vi "Queue - Engine - Main.vi"(6 "timeout in ms (-1)":i32=-1, 7 "Operation":enum16{"Enqueue", "Dequeue", "Flush", "Release"}(ring)=enum."Dequeue", 8 "error in":errorcluster, 10 "Queue Data In":string, 11 "Queue Name In":string) -> (0 "error out":errorcluster, 1 "timed out?":bool, 2 "Data Out":string)   [LabVIEW 2011]
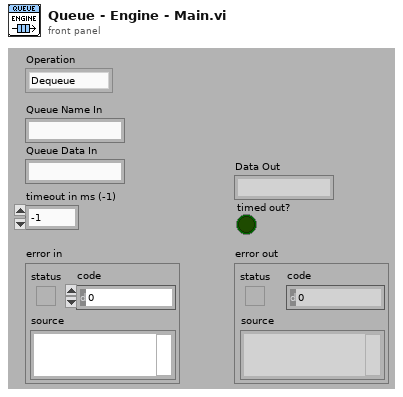
[diagram p1: front panel]
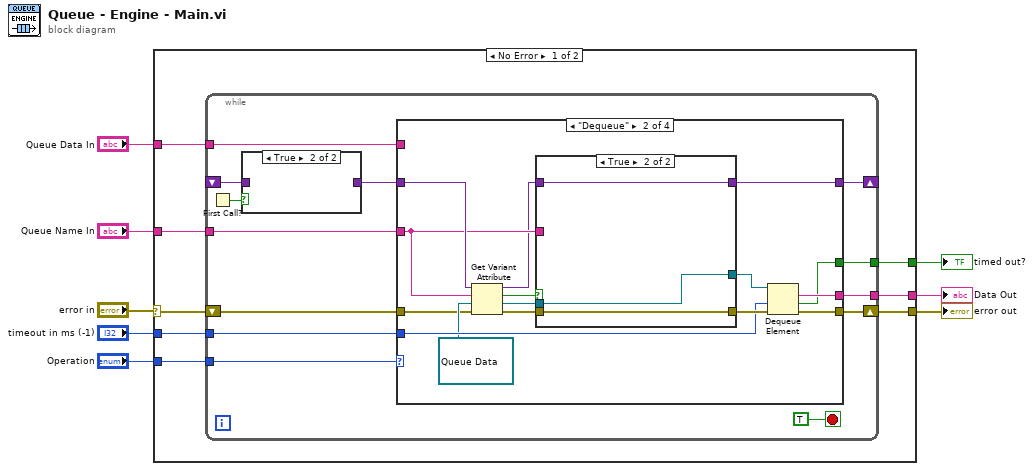
[diagram p0: block diagram]
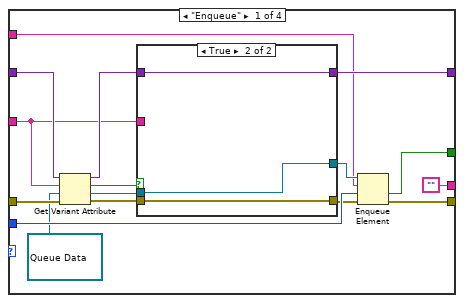
[diagram p3: hidden frame]
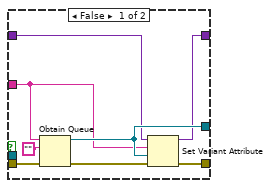
[diagram p4: hidden frame]
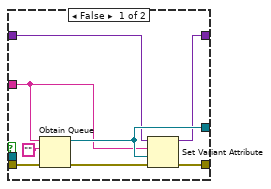
[diagram p5: hidden frame]
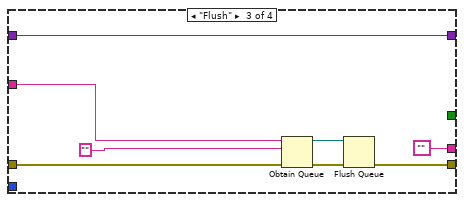
[diagram p6: hidden frame]
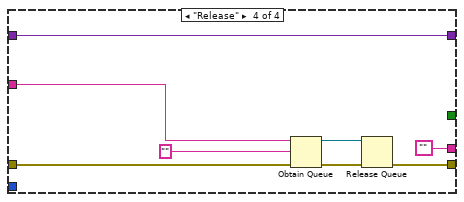
[diagram p7: hidden frame]
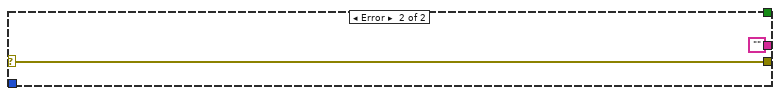
[diagram p8: hidden frame]
diagram:
  n1 = case shown="No Error" "error in" {
    selector: "error in" -> [w12 w101]
    tunnel: "Operation" -> [w16 _]
    tunnel: "Queue Name In" -> [w15 _]
    tunnel: "Queue Data In" -> [w14 _]
    tunnel: [w13 ""] -> w5
    tunnel: [w11 w101] -> w3
    tunnel: "timeout in ms (-1)" -> [w10 _]
    tunnel: [w9 _] -> w1
    frame No Error {
      n2 = while {
        tunnel: w16 -> [w29]
        tunnel: w15 -> [w23]
        shift-right: [w27] -> w11
        shift-left: w12 -> [w26]
        tunnel: [w25] -> w13
        tunnel: w14 -> [w24]
        tunnel: w10 -> [w22]
        tunnel: [w21] -> w9
        shift-right: [w20] -> _
        shift-left: _ -> [w19]
        stop <- TRUE stop-if-true
        n3 = First Call?() -> (First Call?: T/F=w18:bool)
        n4 = case shown="True" w18 {
          tunnel: w19 -> [w30 _]
          tunnel: [w30 _] -> w17
          frame False {
          }
          frame True {
          }
        }
        n5 = case shown="\"Dequeue\"" w29 {
          tunnel: [w46 w71 w87 w97] -> w27
          tunnel: w26 -> [w42 w65 w91 w99]
          tunnel: ["" w69 "" ""] -> w25
          tunnel: w24 -> [w31 _ _ _]
          tunnel: w23 -> [w32 w60 w90 w95]
          tunnel: w22 -> [w44 w68 _ _]
          tunnel: [w43 w67 _ _] -> w21
          tunnel: w17 -> [w41 w63 w84 w92]
          tunnel: [w33 w58 w84 w92] -> w20
          frame "Enqueue" {
            n6 = Get Variant Attribute(Variant=w41, name=w32, default value (empty Variant)=refnum<queue> refnum ("queue out"), error in=w42) -> (duplicate Variant=w34:variant, found=w36:bool, value=w35:refnum<queue>, error out=w37:errorcluster)
            n7 = case shown="True" w36 {
              tunnel: [w52 w57] -> w39
              tunnel: [w50 w56] -> w38
              tunnel: w37 -> [w53 w56]
              tunnel: w35 -> [_ w57]
              tunnel: w32 -> [w48 _]
              tunnel: [w49 w55] -> w33
              tunnel: w34 -> [w47 w55]
              frame False {
                n8 = Obtain Queue(name (unnamed)=w48, element data type="", error in (no error)=w53) -> (queue out=w52:refnum<queue>, error out=w51:errorcluster)  [unwired: 2 in, 1 out]
                n9 = Set Variant Attribute(Variant=w47, name=w48, value=w52, error in=w51) -> (Variant out=w49:variant, error out=w50:errorcluster)  [unwired: 1 out]
              }
              frame True {
              }
            }
            n10 = Enqueue Element(queue=w39, element=w31, timeout in ms (-1)=w44, error in (no error)=w38) -> (timed out?=w43:bool, error out=w46:errorcluster)  [unwired: 1 out]
          }
          frame "Dequeue" {
            n11 = Get Variant Attribute(Variant=w63, name=w60, default value (empty Variant)=refnum<queue> refnum ("queue out"), error in=w65) -> (duplicate Variant=w59:variant, found=w62:bool, value=w61:refnum<queue>, error out=w64:errorcluster)
            n12 = case shown="True" w62 {
              tunnel: [w78 w83] -> w72
              tunnel: [w76 w82] -> w70
              tunnel: w64 -> [w79 w82]
              tunnel: w61 -> [_ w83]
              tunnel: w60 -> [w73 _]
              tunnel: w59 -> [w75 w81]
              tunnel: [w74 w81] -> w58
              frame False {
                n13 = Obtain Queue(name (unnamed)=w73, element data type="", error in (no error)=w79) -> (queue out=w78:refnum<queue>, error out=w77:errorcluster)  [unwired: 2 in, 1 out]
                n14 = Set Variant Attribute(Variant=w75, name=w73, value=w78, error in=w77) -> (Variant out=w74:variant, error out=w76:errorcluster)  [unwired: 1 out]
              }
              frame True {
              }
            }
            n15 = Dequeue Element(queue=w72, timeout in ms (-1)=w68, error in (no error)=w70) -> (element=w69:string, timed out?=w67:bool, error out=w71:errorcluster)  [unwired: 1 out]
          }
          frame "Flush" {
            n16 = Obtain Queue(name (unnamed)=w90, element data type="" ("Queue Name"), error in (no error)=w91) -> (queue out=w86:refnum<queue>, error out=w88:errorcluster)  [unwired: 2 in, 1 out]
            n17 = Flush Queue(queue=w86, error in (no error)=w88) -> (error out=w87:errorcluster)  [unwired: 2 out]
          }
          frame "Release" {
            n18 = Obtain Queue(name (unnamed)=w95, element data type="" ("Queue Data"), error in (no error)=w99) -> (queue out=w96:refnum<queue>, error out=w98:errorcluster)  [unwired: 2 in, 1 out]
            n19 = Release Queue(queue=w96, error in (no error)=w98) -> (error out=w97:errorcluster)  [unwired: 1 in, 2 out]
          }
        }
      }
    }
    frame Error {
    }
  }
  "Data Out" <- w5
  "error out" <- w3
  "timed out?" <- w1
